vi "EOL CAN_Enter Diag Session.vi"(7 "Rx Arbitration Id":u32=402522244 format="%.0x", 8 "Error in":errorcluster, 9 "Session":T1, 10 "Read Session in":refnum<k21>, 11 "Write Session in":refnum<k21>) -> (0 "Error out":errorcluster, 2 "TxRx Data":string[][](array[string]), 3 "Response Good?":bool)   [LabVIEW 2018]
uses:
  Typedefs/Select Session.ctl
  <vilib>/xnet/xnet.llb/XNET Frame CAN.ctl
  <vilib>/xnet/xnet.llb/XNET Frame Type CAN.ctl
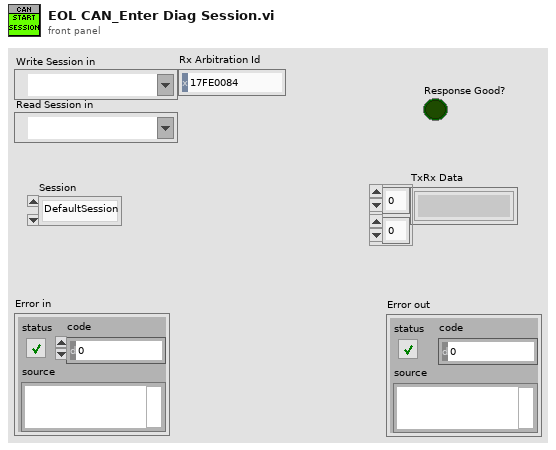
[diagram p1: front panel]
types:
  T1 = typedef "Select Session.ctl" = enum16{"DefaultSession", "Development", "Extended", "EOL", "Programming"}
  T2 = typedef "XNET Frame CAN.ctl" = cluster{"timestamp":timestamp, "payload":u8[], "identifier":u32, "type":T3, "extended?":bool, "echo?":bool}
  T3 = typedef "XNET Frame Type CAN.ctl" = u8
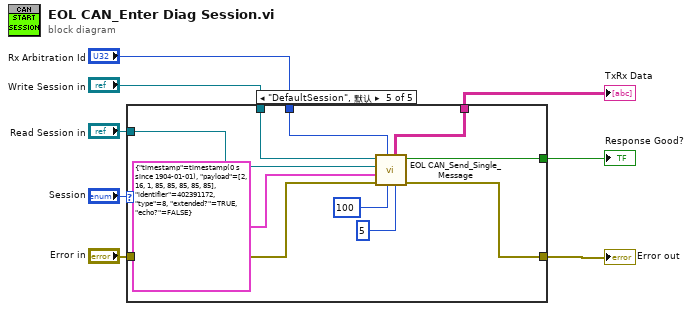
[diagram p0: block diagram]
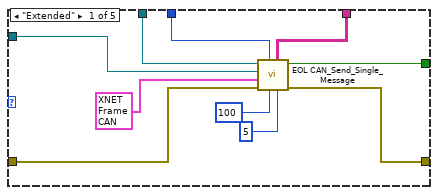
[diagram p2: hidden frame]
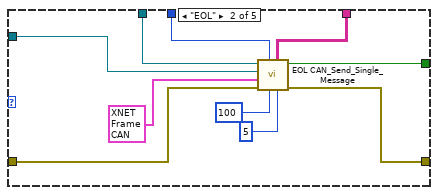
[diagram p3: hidden frame]
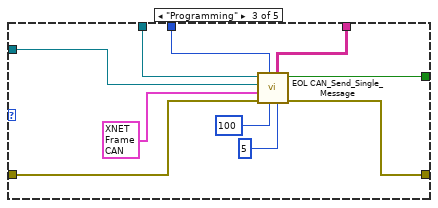
[diagram p4: hidden frame]
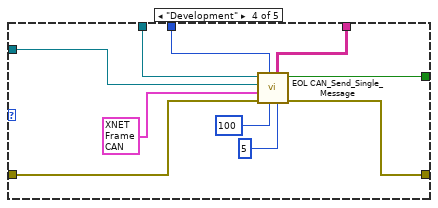
[diagram p5: hidden frame]
diagram:
  n1 = case shown="\"DefaultSession\", 默认" "Session" {
    tunnel: "Error in" -> [w18 w28 w38 w48 w58]
    tunnel: [w17 w27 w37 w47 w57] -> w7
    tunnel: [w16 w26 w36 w46 w56] -> w6
    tunnel: "Rx Arbitration Id" -> [w15 w25 w35 w45 w55]
    tunnel: "Write Session in" -> [w14 w24 w34 w44 w54]
    tunnel: "Read Session in" -> [w13 w23 w33 w43 w53]
    tunnel: [w12 w22 w32 w42 w52] -> w2
    frame "Extended" {
      n2 = call "EOL CAN_Send_Single_Message.vi"("Retries"=5, "Msg Wait Time"=u32 100, "Rx Arbitration Id"=w15, "Error in"=w18, "Tx CAN frame"=T2 {"timestamp"=timestamp(0 s since 1904-01-01), "payload"=[2, 16, 3, 85, 85, 85, 85, 85], "identifier"=402391172, "type"=8, "extended?"=TRUE, "echo?"=FALSE}, "Read Session in"=w13, "Write Session in"=w14) -> ("Error out"=w17:errorcluster, "Response Good?"=w12:bool, "TxRx Data"=w16:string[][])  [unwired: 2 out]
    }
    frame "EOL" {
      n3 = call "EOL CAN_Send_Single_Message.vi"("Retries"=5, "Msg Wait Time"=u32 100, "Rx Arbitration Id"=w25, "Error in"=w28, "Tx CAN frame"=T2 {"timestamp"=timestamp(0 s since 1904-01-01), "payload"=[2, 16, 64, 85, 85, 85, 85, 85], "identifier"=402391172, "type"=8, "extended?"=TRUE, "echo?"=FALSE}, "Read Session in"=w23, "Write Session in"=w24) -> ("Error out"=w27:errorcluster, "Response Good?"=w22:bool, "TxRx Data"=w26:string[][])  [unwired: 2 out]
    }
    frame "Programming" {
      n4 = call "EOL CAN_Send_Single_Message.vi"("Retries"=5, "Msg Wait Time"=u32 100, "Rx Arbitration Id"=w35, "Error in"=w38, "Tx CAN frame"=T2 {"timestamp"=timestamp(0 s since 1904-01-01), "payload"=[2, 16, 2, 85, 85, 85, 85, 85], "identifier"=402391172, "type"=8, "extended?"=TRUE, "echo?"=FALSE}, "Read Session in"=w33, "Write Session in"=w34) -> ("Error out"=w37:errorcluster, "Response Good?"=w32:bool, "TxRx Data"=w36:string[][])  [unwired: 2 out]
    }
    frame "Development" {
      n5 = call "EOL CAN_Send_Single_Message.vi"("Retries"=5, "Msg Wait Time"=u32 100, "Rx Arbitration Id"=w45, "Error in"=w48, "Tx CAN frame"=T2 {"timestamp"=timestamp(0 s since 1904-01-01), "payload"=[2, 16, 79, 85, 85, 85, 85, 85], "identifier"=402391172, "type"=8, "extended?"=TRUE, "echo?"=FALSE}, "Read Session in"=w43, "Write Session in"=w44) -> ("Error out"=w47:errorcluster, "Response Good?"=w42:bool, "TxRx Data"=w46:string[][])  [unwired: 2 out]
    }
    frame "DefaultSession", Default {
      n6 = call "EOL CAN_Send_Single_Message.vi"("Retries"=5, "Msg Wait Time"=u32 100, "Rx Arbitration Id"=w55, "Error in"=w58, "Tx CAN frame"=T2 {"timestamp"=timestamp(0 s since 1904-01-01), "payload"=[2, 16, 1, 85, 85, 85, 85, 85], "identifier"=402391172, "type"=8, "extended?"=TRUE, "echo?"=FALSE}, "Read Session in"=w53, "Write Session in"=w54) -> ("Error out"=w57:errorcluster, "Response Good?"=w52:bool, "TxRx Data"=w56:string[][])  [unwired: 2 out]
    }
  }
  "Error out" <- w7
  "TxRx Data" <- w6
  "Response Good?" <- w2
